vi "OTP TESTBENCH.vi"() -> ()   [LabVIEW 2013]
panel:
  out "result":u8[](array[numeric])
  out "message":u8[](array[numeric])
  out "original message":string
  out "ciphertext (Public)":string
  out "Key (Private)":string
  in  "ASCII":cluster{i32, string}[](array[cluster])=[{0, "\u0000"}, {1, "\u0001"}, {2, "\u0002"}, {3, "\u0003"}, {4, "\u0004"}, {5, "\u0005"}, {6, "\u0006"}, {7, "\u0007"}, {8, "\b"}, {9, "\t"}, {10, "\n"}, {11, "\u000b"}, {12, "\f"}, {13, "\r"}, {14, "\u000e"}, {15, "\u000f"}, {16, "\u0010"}, {17, "\u0011"}, {18, "\u0012"}, {19, "\u0013"}, {20, "\u0014"}, {21, "\u0015"}, {22, "\u0016"}, {23, "\u0017"}, {24, "\u0018"}, {25, "\u0019"}, {26, "\u001a"}, {27, "\u001b"}, {28, "\u001c"}, {29, "\u001d"}, {30, "\u001e"}, {31, "\u001f"}, {32, " "}, {33, "!"}, {34, "\""}, {35, "#"}, {36, "$"}, {37, "%"}, {38, "&"}, {39, "'"}, {40, "("}, {41, ")"}, {42, "*"}, {43, "+"}, {44, ","}, {45, "-"}, {46, "."}, {47, "/"}, {48, "0"}, {49, "1"}, {50, "2"}, {51, "3"}, {52, "4"}, {53, "5"}, {54, "6"}, {55, "7"}, {56, "8"}, {57, "9"}, {58, ":"}, {59, ";"}, {60, "<"}, {61, "="}, {62, ">"}, {63, "?"}, {64, "@"}, {65, "A"}, {66, "B"}, {67, "C"}, {68, "D"}, {69, "E"}, {70, "F"}, {71, "G"}, {72, "H"}, {73, "I"}, {74, "J"}, {75, "K"}, {76, "L"}, {77, "M"}, {78, "N"}, {79, "O"}, {80, "P"}, {81, "Q"}, {82, "R"}, {83, "S"}, {84, "T"}, {85, "U"}, {86, "V"}, {87, "W"}, {88, "X"}, {89, "Y"}, {90, "Z"}, {91, "["}, {92, "\\"}, {93, "]"}, {94, "^"}, {95, "_"}, {96, "`"}, {97, "a"}, {98, "b"}, {99, "c"}, {100, "d"}, {101, "e"}, {102, "f"}, {103, "g"}, {104, "h"}, {105, "i"}, {106, "j"}, {107, "k"}, {108, "l"}, {109, "m"}, {110, "n"}, {111, "o"}, {112, "p"}, {113, "q"}, {114, "r"}, {115, "s"}, {116, "t"}, {117, "u"}, {118, "v"}, {119, "w"}, {120, "x"}, {121, "y"}, {122, "z"}, {123, "{"}, {124, "|"}, {125, "}"}, {126, "~"}, {127, ""}, {128, "€"}, {129, ""}, {130, "‚"}, {131, "ƒ"}, {132, "„"}, {133, "…"}, {134, "†"}, {135, "‡"}, {136, "ˆ"}, {137, "‰"}, {138, "Š"}, {139, "‹"}, {140, "Œ"}, {141, ""}, {142, "Ž"}, {143, ""}, {144, ""}, {145, "‘"}, {146, "’"}, {147, "“"}, {148, "”"}, {149, "•"}, {150, "–"}, {151, "—"}, {152, "˜"}, {153, "™"}, {154, "š"}, {155, "›"}, {156, "œ"}, {157, ""}, {158, "ž"}, {159, "Ÿ"}, {160, " "}, {161, "¡"}, {162, "¢"}, {163, "£"}, {164, "¤"}, {165, "¥"}, {166, "¦"}, {167, "§"}, {168, "¨"}, {169, "©"}, {170, "ª"}, {171, "«"}, {172, "¬"}, {173, "­"}, {174, "®"}, {175, "¯"}, {176, "°"}, {177, "±"}, {178, "²"}, {179, "³"}, {180, "´"}, {181, "µ"}, {182, "¶"}, {183, "·"}, {184, "¸"}, {185, "¹"}, {186, "º"}, {187, "»"}, {188, "¼"}, {189, "½"}, {190, "¾"}, {191, "¿"}, {192, "À"}, {193, "Á"}, {194, "Â"}, {195, "Ã"}, {196, "Ä"}, {197, "Å"}, {198, "Æ"}, {199, "Ç"}, {200, "È"}, {201, "É"}, {202, "Ê"}, {203, "Ë"}, {204, "Ì"}, {205, "Í"}, {206, "Î"}, {207, "Ï"}, {208, "Ð"}, {209, "Ñ"}, {210, "Ò"}, {211, "Ó"}, {212, "Ô"}, {213, "Õ"}, {214, "Ö"}, {215, "×"}, {216, "Ø"}, {217, "Ù"}, {218, "Ú"}, {219, "Û"}, {220, "Ü"}, {221, "Ý"}, {222, "Þ"}, {223, "ß"}, {224, "à"}, {225, "á"}, {226, "â"}, {227, "ã"}, {228, "ä"}, {229, "å"}, {230, "æ"}, {231, "ç"}, {232, "è"}, {233, "é"}, {234, "ê"}, {235, "ë"}, {236, "ì"}, {237, "í"}, {238, "î"}, {239, "ï"}, {240, "ð"}, {241, "ñ"}, {242, "ò"}, {243, "ó"}, {244, "ô"}, {245, "õ"}, {246, "ö"}, {247, "÷"}, {248, "ø"}, {249, "ù"}, {250, "ú"}, {251, "û"}, {252, "ü"}, {253, "ý"}, {254, "þ"}, {255, "ÿ"}]
  in  "Message":string
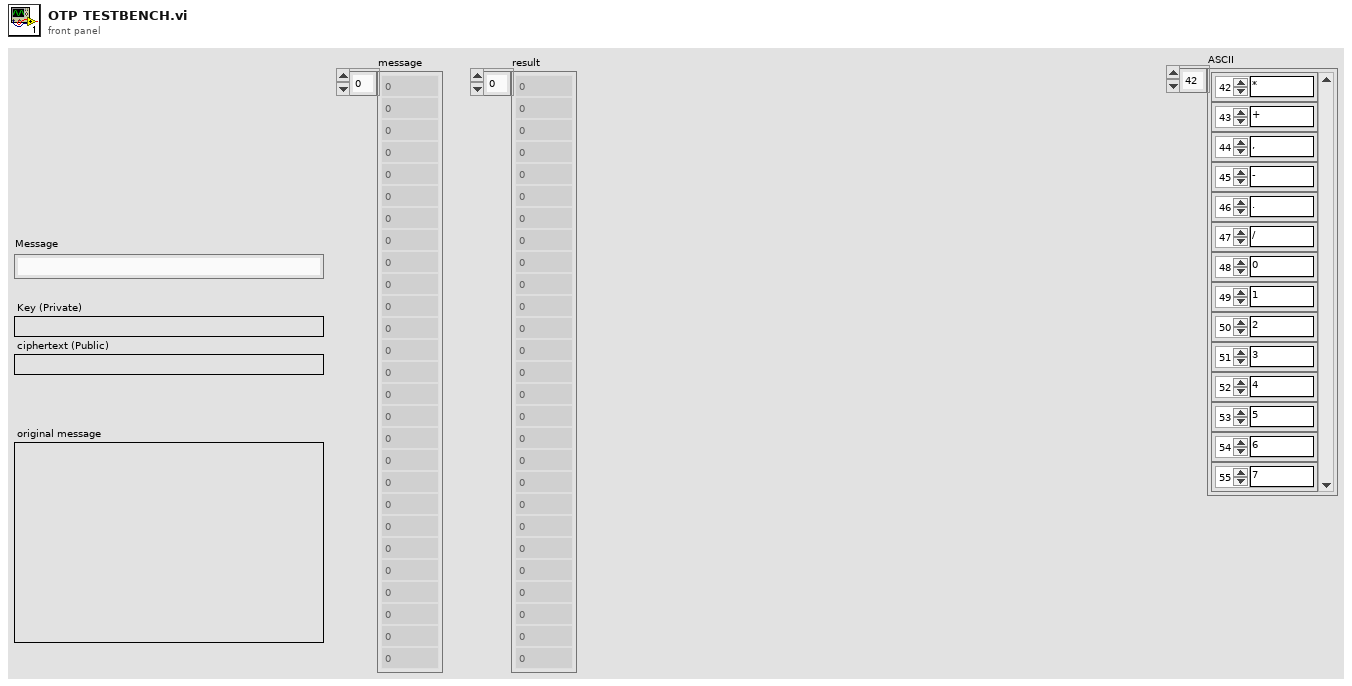
[diagram p1: front panel]
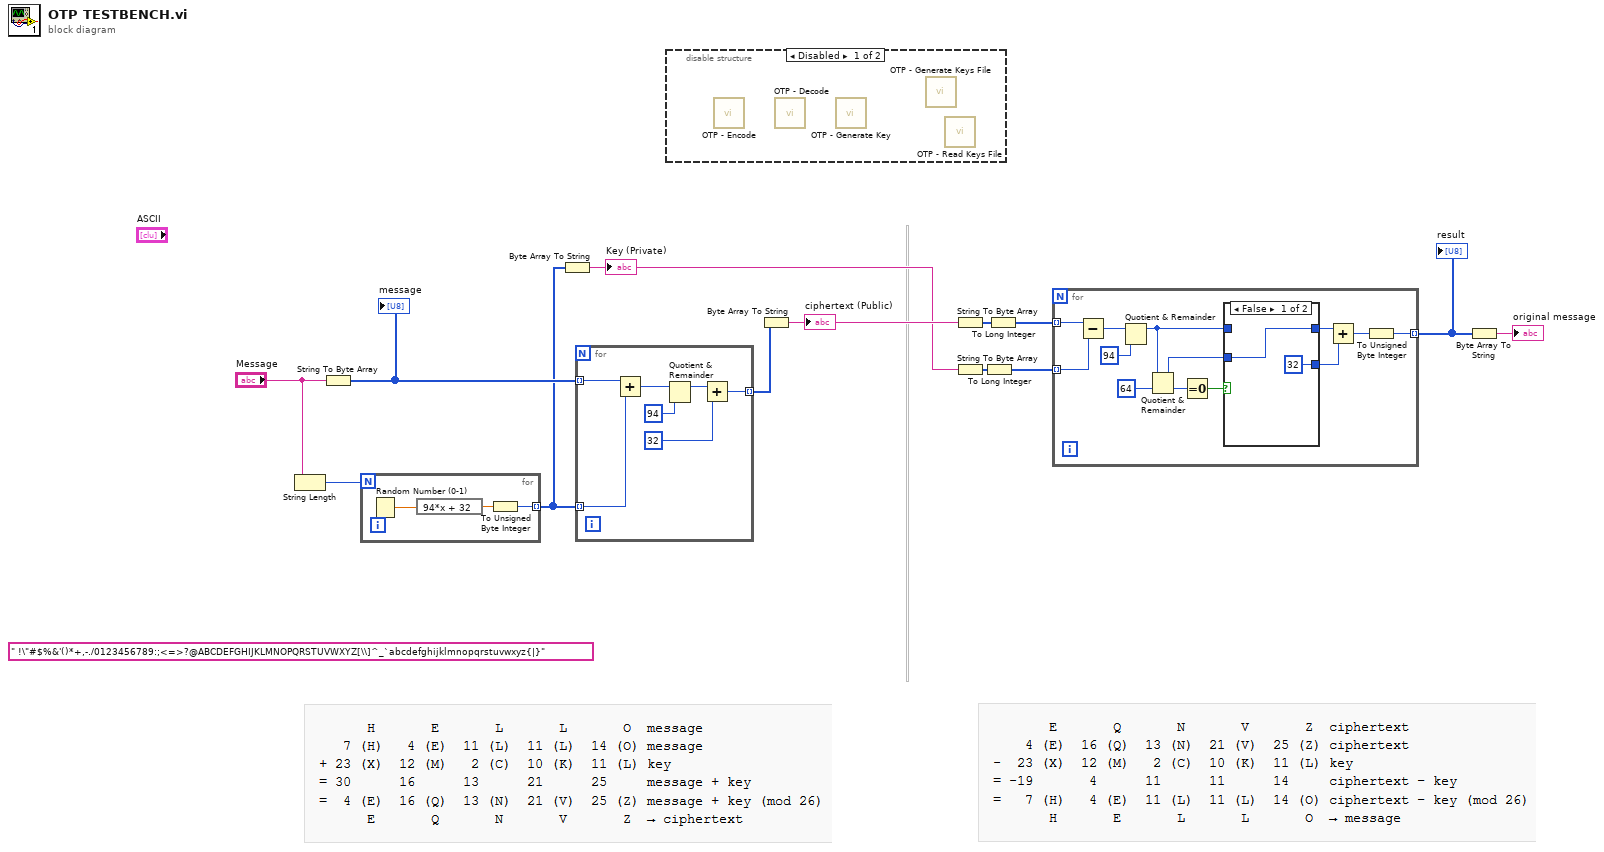
[diagram p0: block diagram]
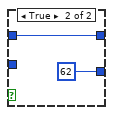
[diagram p3: hidden frame]
diagram:
  (unwired) " !\"#$%&'()*+,-./0123456789:;<=>?@ABCDEFGHIJKLMNOPQRSTUVWXYZ[\\]^_`abcdefghijklmnopqrstuvwxyz{|}" ("String")
  n1 = String Length(string="Message") -> (length=w13:i32)
  n2 = String To Byte Array(string="Message") -> (unsigned byte array=w12:u8[])
  "message" <- w12
  n3 = for {
    N: w13 -> [_]
    tunnel: [w14] -> w11 mode=indexing
    n4 = Random Number (0-1)() -> (number: 0 to 1=w16:dbl)
    n5 = expression code="94*x + 32"(w16) -> (w15:dbl)
    n6 = To Unsigned Byte Integer(number=w15) -> (unsigned 8bit integer=w14:u8)
  }
  n7 = Byte Array To String(unsigned byte array=w11) -> (string=w9:string)
  "Key (Private)" <- w9
  n8 = for {
    tunnel: w12 -> [w23] mode=indexing
    tunnel: w11 -> [w22] mode=indexing
    tunnel: [w19] -> w5 mode=indexing
    n9 = Add(x=w23, y=w22) -> (x+y=w21:u8)
    n10 = Quotient & Remainder(x=w21, y=u8 94) -> (x-y*floor(x/y)=w17:u8)  [unwired: 1 out]
    n11 = Add(x=w17, y=u8 32) -> (x+y=w19:u8)
  }
  n12 = disable-structure shown="Disabled" {
    frame Disabled {
      n13 = call "OTP - Encode.vi"() -> ()  [unwired: 11 in, 1 out]
      n14 = call "OTP - Decode.vi"() -> ()  [unwired: 11 in, 1 out]
      n15 = call "OTP - Generate Key.vi"() -> ()  [unwired: 11 in, 1 out]
      n16 = call "OTP - Generate Keys File.vi"() -> ()  [unwired: 12 in]
      n17 = call "OTP - Read Keys File.vi"() -> ()  [unwired: 11 in, 1 out]
    }
    frame Enabled {
    }
  }
  n18 = Byte Array To String(unsigned byte array=w5) -> (string=w10:string)
  "ciphertext (Public)" <- w10
  n19 = String To Byte Array(string=w10) -> (unsigned byte array=w7:u8[])
  n20 = String To Byte Array(string=w9) -> (unsigned byte array=w8:u8[])
  n21 = To Long Integer(number=w8) -> (32bit integer=w3:i32[])
  n22 = To Long Integer(number=w7) -> (32bit integer=w4:i32[])
  n23 = for {
    tunnel: w3 -> [w35] mode=indexing
    tunnel: w4 -> [w36] mode=indexing
    tunnel: [w33] -> w6 mode=indexing
    n24 = Subtract(x=w36, y=w35) -> (x-y=w31:i32)
    n25 = Quotient & Remainder(x=w31, y=94) -> (x-y*floor(x/y)=w26:i32)  [unwired: 1 out]
    n26 = Quotient & Remainder(x=w26, y=64) -> (x-y*floor(x/y)=w27:i32, floor(x/y)=w29:i32)
    n27 = Equal To 0?(x=w29) -> (x = 0?=w28:bool)
    n28 = case shown="False" w28 {
      tunnel: w27 -> [w37 _]
      tunnel: w26 -> [_ w40]
      tunnel: [w37 w40] -> w25
      tunnel: [32 ("y") 62 ("y")] -> w24
      frame False {
      }
      frame True {
      }
    }
    n29 = Add(x=w25, y=w24) -> (x+y=w32:i32)
    n30 = To Unsigned Byte Integer(number=w32) -> (unsigned 8bit integer=w33:u8)
  }
  "result" <- w6
  n31 = Byte Array To String(unsigned byte array=w6) -> (string=→"original message":string)
